vi "Convert_data_read_to_speed.vi"(1 "Byte Array":u8[](array[numeric])) -> (0 "Speed":i16)   [LabVIEW 2019]
doc: "This vi converts value read for \"Read_Real_Speed_Command.vi\" to a speed value in RPM."
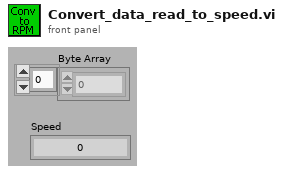
[diagram p1: front panel]
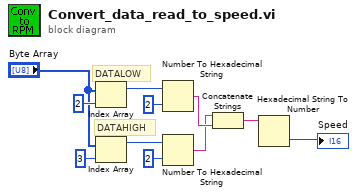
[diagram p0: block diagram]
diagram:
  # "DATAHIGH"
  # "DATALOW"
  n1 = Index Array(array="Byte Array", index=2 ("Index")) -> (element=w6:u8)
  n2 = Index Array(array="Byte Array", index=3 ("Index")) -> (element=w7:u8)
  n3 = Number To Hexadecimal String(1:i16 2 ("width (-)"), 2:w6) -> (0:w5:string)
  n4 = Number To Hexadecimal String(1:i16 2 ("width (-)"), 2:w7) -> (0:w4:string)
  n5 = Concatenate Strings(w4, w5) -> (w3:string)
  n6 = Hexadecimal String To Number(string=w3) -> (number=→"Speed":u32)  [unwired: 2 in, 1 out]
